vi "InsertRectangle.vi"(8 "SquuareSide":i32, 9 "Top":i32, 10 "Left":i32, 11 "Refnum in":T1) -> (3 "Refnum out":T1)   [LabVIEW 2015]
uses:
  <vilib>/vision/Image Controls.llb/IMAQ Image.ctl
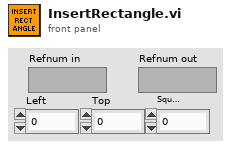
[diagram p1: front panel]
types:
  T1 = typedef "IMAQ Image.ctl" = refnum<image>
  T2 = cluster{"Left":i32, "Top":i32, "Right":i32, "Bottom":i32}
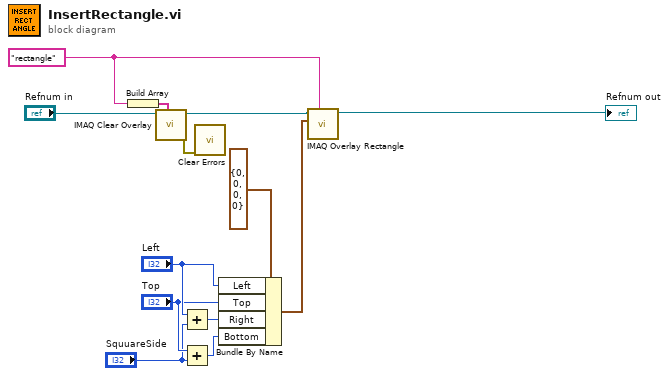
[diagram p0: block diagram]
diagram:
  w3 = "rectangle" ("Group")
  n1 = Build Array(w3) -> (w2:string[])
  n2 = call "IMAQ Clear Overlay"("Groups"=w2, "Image"="Refnum in") -> ("error out"=w1:errorcluster, "Image Out"=w4:T1)  [unwired: 8 in]
  n3 = Add(x="Left", y="SquuareSide") -> (x+y=w8:i32)
  n4 = Add(x="Top", y="SquuareSide") -> (x+y=w5:i32)
  n5 = call <vilib>:"Clear Errors.vi"("error in (no error)"=w1) -> ()  [unwired: 5 in, 2 out]
  n6 = Bundle By Name(cluster=T2 {"Left"=0, "Top"=0, "Right"=0, "Bottom"=0} ("Rectangle"), "Left"="Left", "Top"="Top", "Right"=w8, "Bottom"=w5) -> (w10:T2)
  n7 = call "IMAQ Overlay Rectangle"("Group"=w3, "Rectangle"=w10, "Image"=w4) -> ("Image Out"=→"Refnum out":T1)  [unwired: 7 in, 1 out]
